vi "Process_Trace.vi"(0 "Channel 1?":bool, 1 "Data in":u8[](array[numeric]), 5 "Length":i32, 12 "Data_Filter":T2 caption="Filter", 13 "M-Thresholds":T1 {"Ch1_Thres_Low" min=-2500.0 max=0.0 scale=0.0..-2500.0 scale format="%#.1f"; "Ch1_Thres_High" min=-2500.0 max=0.0 scale=0.0..-2500.0 scale format="%#.1f"; "Ch2_Thres_High" min=-2500.0 max=0.0 scale=0.0..-2500.0 scale format="%#.1f"; "Ch2_Thres_Low" min=-2500.0 max=0.0 scale=0.0..-2500.0 scale format="%#.1f"}) -> (2 "Standard deviation":i16, 3 "Data out":u8[](array[numeric]), 4 "Baseline":i16, 6 "Number of peaks":i16, 8 "Pulse height":i16, 10 "Integral":i32, 14 "Offset":i16, 15 "Cut off":i16)   [LabVIEW 2013]
uses:
  Controls/TabPage_Thresholds.ctl
panel:
  out "size(s) 2":i32
  out "size(s)":i32
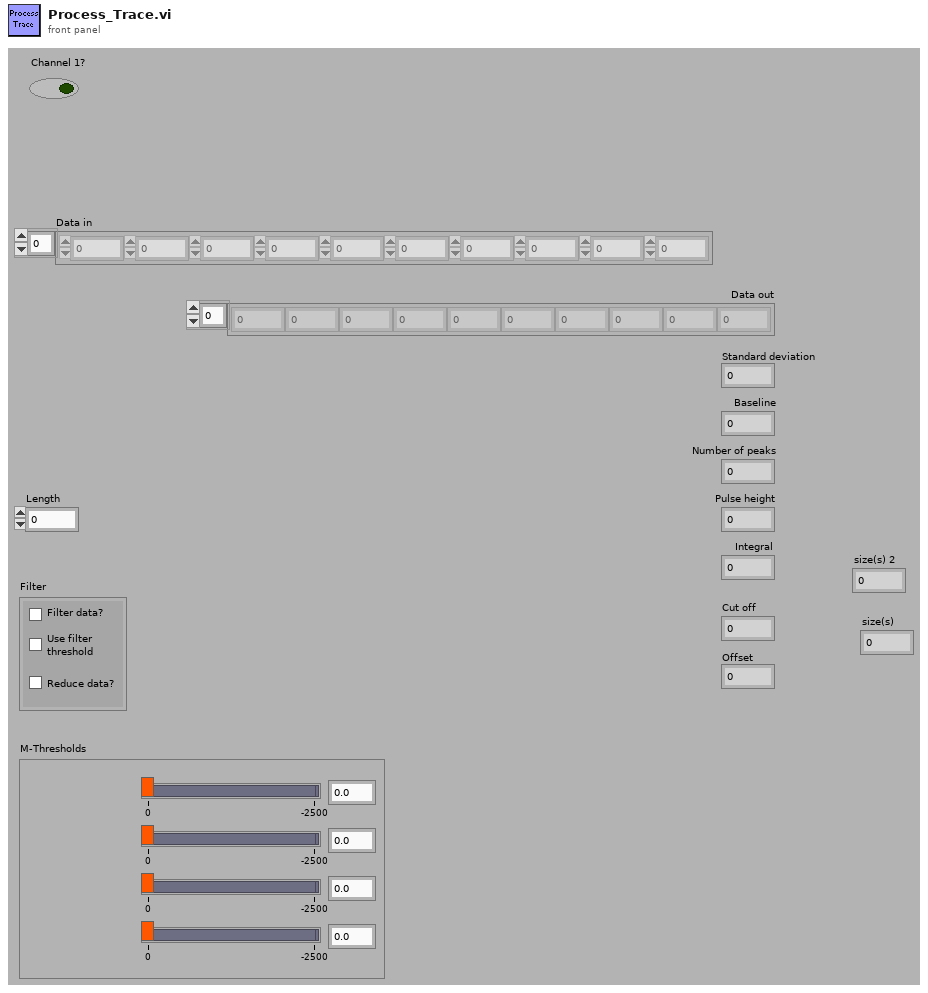
[diagram p1: front panel]
types:
  T1 = typedef "TabPage_Thresholds.ctl" = cluster{"Ch1_Thres_Low":dbl, "Ch1_Thres_High":dbl, "Ch2_Thres_Low":dbl, "Ch2_Thres_High":dbl}
  T2 = cluster{"Filter_Data":bool, "Use_Thresh":bool, "Reduce data?":bool}
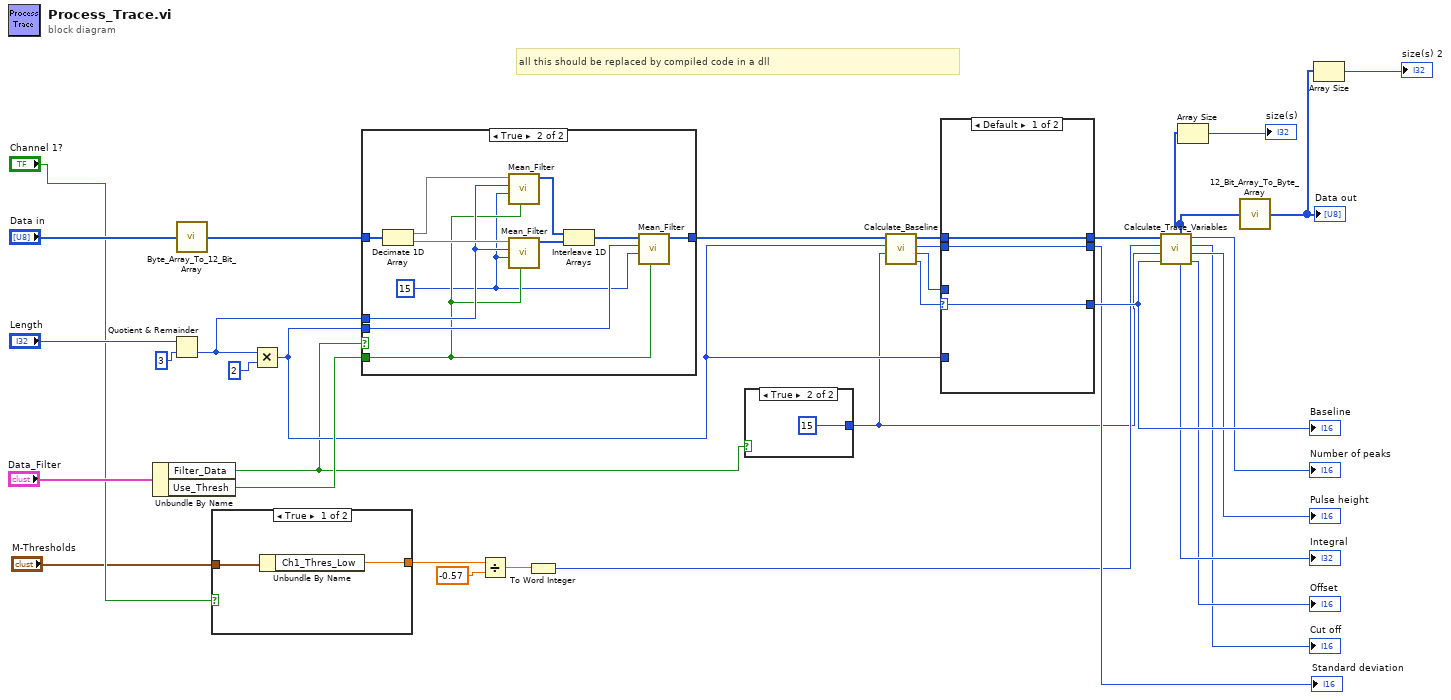
[diagram p0: block diagram]
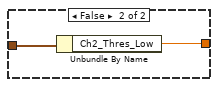
[diagram p2: hidden frame]
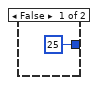
[diagram p3: hidden frame]
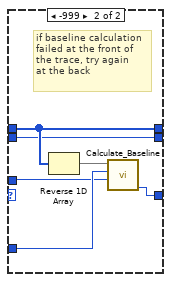
[diagram p5: hidden frame]
diagram:
  # "all this should be replaced by compiled code in a dll"
  n1 = Unbundle By Name("Data_Filter") -> ("Filter_Data"=w14:bool, "Use_Thresh"=w34:bool)
  n2 = Quotient & Remainder(x="Length", y=3) -> (floor(x/y)=w33:i32)  [unwired: 1 out]
  n3 = call "Byte_Array_To_12_Bit_Array.vi"("Byte-Array"="Data in") -> ("12-Bit-Array"=w27:u16[])
  n4 = case shown="True" "Channel 1?" {
    tunnel: "M-Thresholds" -> [w36 w38]
    tunnel: [w35 w37] -> w10
    frame True {
      n5 = Unbundle By Name(w36) -> ("Ch1_Thres_Low"=w35:dbl)
    }
    frame False {
      n6 = Unbundle By Name(w38) -> ("Ch2_Thres_Low"=w37:dbl)
    }
  }
  n7 = Multiply(x=w33, y=2) -> (x*y=w29:i32)
  n8 = case shown="True" w14 {
    tunnel: w27 -> [w39 w50]
    tunnel: [w39 w44] -> w28
    tunnel: w33 -> [_ w43]
    tunnel: w29 -> [_ w42]
    tunnel: w34 -> [_ w41]
    frame False {
    }
    frame True {
      w40 = u16 15 ("Threshold")
      n9 = Decimate 1D Array(w50) -> (w49:u16[], w46:u16[])
      n10 = call "Mean_Filter.vi"("Filter with threshold?"=w41, "Threshold"=w40, "Length"=w43, "Data in"=w49) -> ("Data out"=w48:u16[])  [unwired: 1 in, 6 out]
      n11 = call "Mean_Filter.vi"("Filter with threshold?"=w41, "Threshold"=w40, "Length"=w43, "Data in"=w46) -> ("Data out"=w47:u16[])  [unwired: 1 in, 6 out]
      n12 = Interleave 1D Arrays(w48, w47) -> (w45:u16[])
      n13 = call "Mean_Filter.vi"("Filter with threshold?"=w41, "Threshold"=w40, "Length"=w42, "Data in"=w45) -> ("Data out"=w44:u16[])  [unwired: 1 in, 6 out]
    }
  }
  n14 = Divide(x=w10, y=-0.57) -> (x/y=w8:dbl)
  n15 = To Word Integer(number=w8) -> (16bit integer=w7:i16)
  n16 = case shown="True" w14 {
    tunnel: [u16 25 ("Threshold in") u16 15 ("Threshold in")] -> w5
    frame False {
    }
    frame True {
    }
  }
  n17 = call "Calculate_Baseline.vi"("Threshold in"=w5, "Length"=w29, "Data in"=w28) -> ("Baseline"=w30:i16, "Threshold out"=w6:u16, "Standard deviation"=w21:i16, "Data out"=w25:u16[])  [unwired: 5 out]
  n18 = case shown="Default" w30 {
    selector: w30 -> [w54 _]
    tunnel: w25 -> [w55 w60]
    tunnel: [w55 w60] -> w32
    tunnel: [w54 w58] -> w31
    tunnel: w29 -> [_ w59]
    tunnel: w21 -> [w53 w57]
    tunnel: [w53 w57] -> w13
    tunnel: w6 -> [_ w56]
    frame Default {
    }
    frame -999 {
      # "if baseline calculation\nfailed at the front of\nthe trace, try again\nat the back"
      n19 = Reverse 1D Array(array=w60) -> (reversed array=w61:u16[])
      n20 = call "Calculate_Baseline.vi"("Threshold in"=w56, "Length"=w59, "Data in"=w61) -> ("Baseline"=w58:i16)  [unwired: 8 out]
    }
  }
  "Baseline" <- w31
  "Standard deviation" <- w13
  n21 = call "Calculate_Trace_Variables.vi"("Baseline"=w31, "Threshold"=w5, "Peak threshold"=w7, "Data in"=w32) -> ("Offset"=→"Offset":i16, "Pulse height"=→"Pulse height":i16, "Cut off"=→"Cut off":i16, "Number of peaks"=→"Number of peaks":i16, "Integral"=→"Integral":i32, "Data out"=w2:u16[])  [unwired: 2 out]
  n22 = Array Size(array=w2) -> (size(s)=→"size(s)":i32)
  n23 = call "12_Bit_Array_To_Byte_Array.vi"("12-Bit-Array"=w2) -> ("Byte-Array"=w1:u8[])
  "Data out" <- w1
  n24 = Array Size(array=w1) -> (size(s)=→"size(s) 2":i32)
